vi "ROI entry-Previous ROI compat_additional.vi"(8 "error in (no error)":errorcluster, 11 "Old ROI file path":path) -> (0 "error out":errorcluster, 1 "Proceed":bool, 3 "Old ROI file path (dup)":path, 5 "ROI fit info cluster":T1 {"ROI fit info"."Frame size"."Old" items=["100X100"=100, "128X128"=128, "200X200"=200, "256X256"=256, "512X512"=512, "1024x1024"=1024, "2048x2048"=2048]; "ROI fit info"."Frame size"."New" items=["100X100"=100, "128X128"=128, "200X200"=200, "256X256"=256, "512X512"=512, "1024x1024"=1024, "2048x2048"=2048]})   [LabVIEW 2017]
uses:
  Typedefs/ROI fitting info cluster.ctl
  Typedefs/Frame Size.ctl
panel:
  in  "Subpanel call":bool
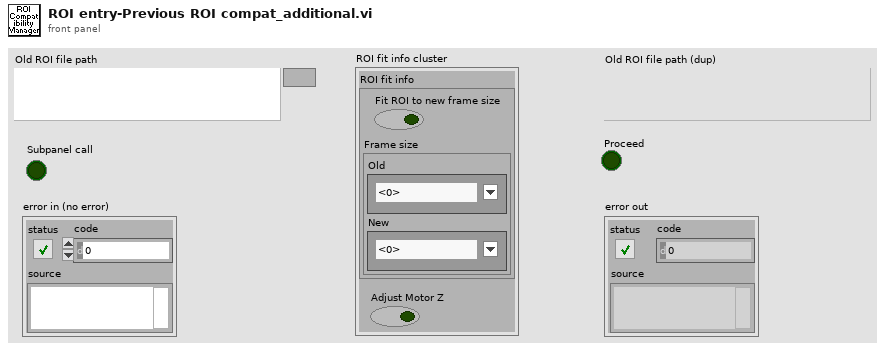
[diagram p1: front panel]
types:
  T1 = typedef "ROI fitting info cluster.ctl" = cluster{"ROI fit info":cluster{"Fit ROI to new frame size":bool, "Frame size":cluster{"Old":T2, "New":T2}}, "Adjust Motor Z":bool}
  T2 = typedef "Frame Size.ctl" = u16
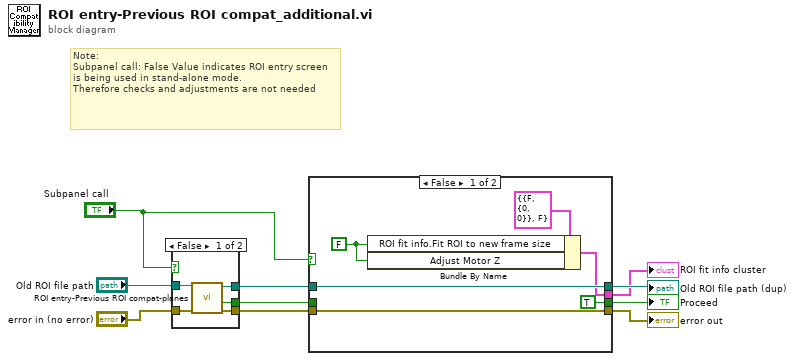
[diagram p0: block diagram]
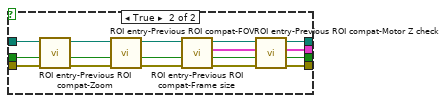
[diagram p2: hidden frame]
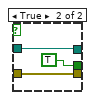
[diagram p3: hidden frame]
diagram:
  # "Note: \nSubpanel call: False Value indicates ROI entry screen is being used in stand-alone mode. \nTherefore checks and adjustments are not needed"
  n1 = case shown="False" "Subpanel call" {
    tunnel: "error in (no error)" -> [w15 w16]
    tunnel: "Old ROI file path" -> [w14 w18]
    tunnel: [w13 w16] -> w8
    tunnel: [w12 TRUE ("Proceed")] -> w7
    tunnel: [w11 w18] -> w6
    frame False {
      n2 = call "ROI entry-Previous ROI compat-planes.vi"("error in (no error)"=w15, "Old ROI file path"=w14) -> ("error out"=w13:errorcluster, "Proceed"=w12:bool, "Old ROI file path (dup)"=w11:path)  [unwired: 7 in]
    }
    frame True {
    }
  }
  n3 = case shown="False" "Subpanel call" {
    tunnel: w8 -> [w23 w41]
    tunnel: w7 -> [_ w40]
    tunnel: w6 -> [w24 w39]
    tunnel: [w24 w37] -> w5
    tunnel: [w23 w35] -> w4
    tunnel: [TRUE ("Proceed") w33] -> w3
    tunnel: [w20 w32] -> w2
    frame False {
      w19 = FALSE
      n4 = Bundle By Name(cluster=T1 {"ROI fit info"={"Fit ROI to new frame size"=FALSE, "Frame size"={"Old"=0, "New"=0}}, "Adjust Motor Z"=FALSE} ("ROI fit info cluster"), "ROI fit info.Fit ROI to new frame size"=w19, "Adjust Motor Z"=w19) -> (w20:T1)
    }
    frame True {
      n5 = call "ROI entry-Previous ROI compat-Zoom.vi"("error in (no error)"=w41, "Proceed"=w40, "Old ROI file path"=w39) -> ("error out"=w30:errorcluster, "Proceed"=w28:bool, "Old ROI file path (dup)"=w26:path)  [unwired: 6 in]
      n6 = call "ROI entry-Previous ROI compat-FOV.vi"("error in (no error)"=w30, "Proceed"=w28, "Old ROI file path"=w26) -> ("error out"=w29:errorcluster, "Proceed"=w27:bool, "Old ROI file path (dup)"=w25:path)  [unwired: 6 in]
      n7 = call "ROI entry-Previous ROI compat-Frame size.vi"("error in (no error)"=w29, "Proceed"=w27, "Old ROI file path"=w25) -> ("error out"=w36:errorcluster, "Proceed"=w34:bool, "ROI fit info"=w31:T1, "Old ROI file path (dup)"=w38:path)  [unwired: 5 in]
      n8 = call "ROI entry-Previous ROI compat-Motor Z check.vi"("error in (no error)"=w36, "Proceed"=w34, "ROI fit info cluster in"=w31, "Old ROI file path"=w38) -> ("error out"=w35:errorcluster, "Proceed"=w33:bool, "ROI fit info cluster"=w32:T1, "Old ROI file path (dup)"=w37:path)  [unwired: 4 in]
    }
  }
  "Proceed" <- w3
  "error out" <- w4
  "Old ROI file path (dup)" <- w5
  "ROI fit info cluster" <- w2
